vi "GW_UW .vi"(8 "error in (no error)":errorcluster, 9 "[glue_workspace_id]":i16=2, 10 "[glue_data_id]":string, 11 "DBlink":string="Driver={ODBC Driver 17 for SQL Server};Server=localhost\\SQLEXPRESS;Database=ZDX201;UID=labview;PWD=Dsa@54137926") -> (0 "error out":errorcluster)   [LabVIEW 2019]
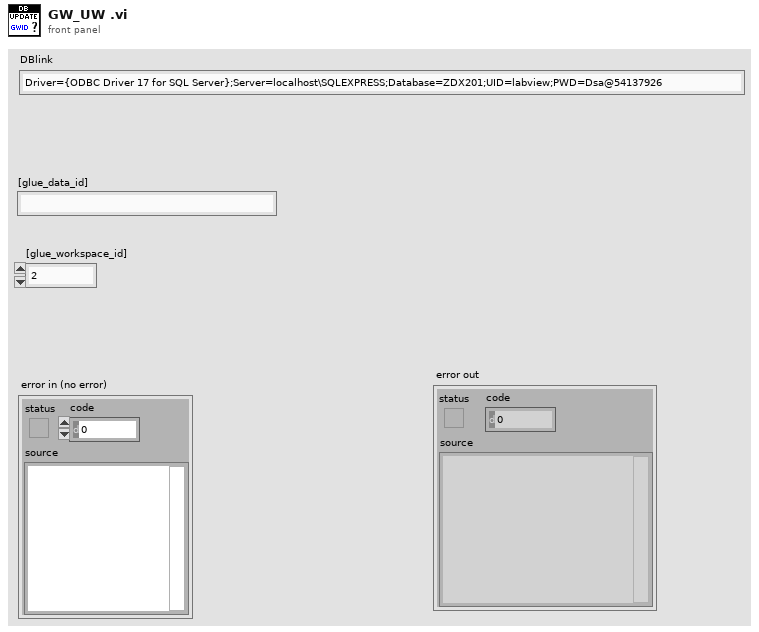
[diagram p1: front panel]
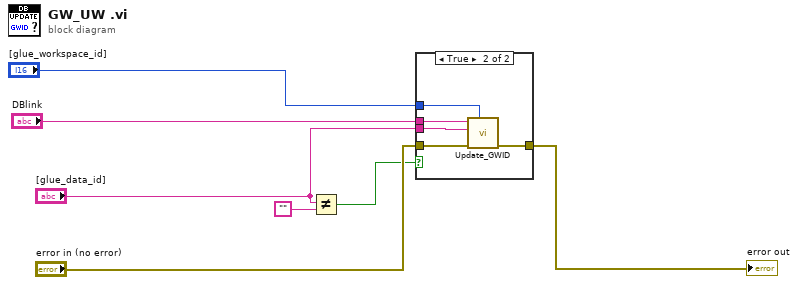
[diagram p0: block diagram]
diagram:
  n1 = Not Equal?(x="[glue_data_id]", y="") -> (x != y?=w2:bool)
  n2 = case shown="True" w2 {
    tunnel: "[glue_workspace_id]" -> [_ w13]
    tunnel: "DBlink" -> [_ w12]
    tunnel: "error in (no error)" -> [w8 w11]
    tunnel: [w8 w10] -> w1
    tunnel: "[glue_data_id]" -> [_ w9]
    frame False {
    }
    frame True {
      n3 = call "Update_GWID .vi"("[glue_workspace_id]"=w13, "error in (no error)"=w11, "[glue_data_id]"=w9, "DBlink"=w12) -> ("error out"=w10:errorcluster)  [unwired: 7 in]
    }
  }
  "error out" <- w1
